vi "Read configuration.vi"(8 "error in":errorcluster, 11 "WaveformAcq editor node in":refnum<class "WaveformAcq editor node.lvclass">) -> (0 "error out":errorcluster, 2 "configuration":refnum<class "NISE_CEF_serializable configuration.lvclass">, 3 "WaveformAcq editor node out":refnum<class "WaveformAcq editor node.lvclass">)   [LabVIEW 2017, in "WaveformAcq editor node.lvclass"]
uses:
  WaveformAcq editor node.lvclass
  <vilib>/NI/Configuration Framework/serializable configuration/NISE_CEF_serializable configuration.lvclass
  WaveformAcq editor node.lvclass/WaveformAcq editor node.ctl
  module/configuration/WaveformAcq configuration.lvclass
  C:/Program Files (x86)/National Instruments/LabVIEW 2017/vi.lib/NI/Configuration Framework/serializable configuration/NISE_CEF_serializable configuration.lvclass
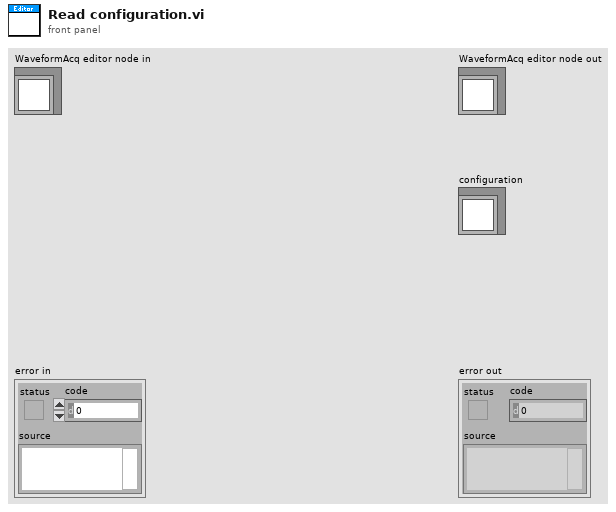
[diagram p1: front panel]
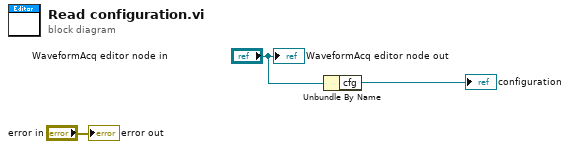
[diagram p0: block diagram]
diagram:
  n1 = Unbundle By Name("WaveformAcq editor node in") -> ("cfg"=→"configuration":refnum<class "WaveformAcq configuration.lvclass">)
  "error out" <- "error in"
  "WaveformAcq editor node out" <- "WaveformAcq editor node in"
